vi "Telescope Move to RA and DEC.vi"(8 "error in (no error)":errorcluster, 10 "Object out":T1, 11 "Telescope in":refnum<class "Telescope.lvclass">) -> (0 "error out":errorcluster, 3 "Telescope out":refnum<class "Telescope.lvclass">)   [LabVIEW 2021, in "Telescope.lvclass"]
uses:
  Telescope.lvclass
  typedefs/CC cluster Object.ctl
  typedefs/CC cluster sidereal rate.ctl
  typedefs/CC cluster RA and DEC.ctl
  typedefs/cc cluster muRA muDEC.ctl
  CC cluster Telescope Offsets.ctl
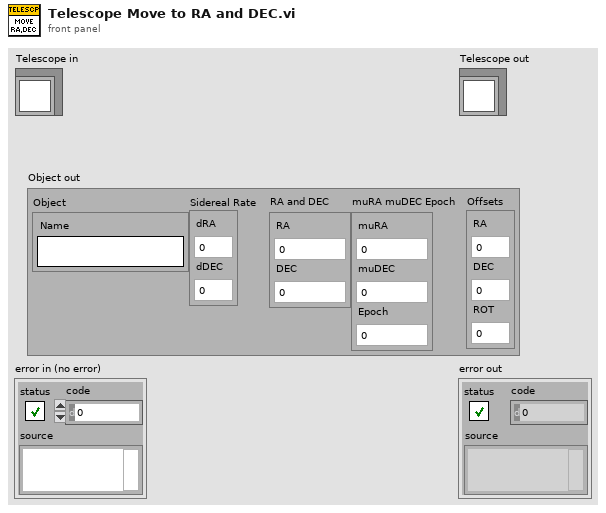
[diagram p1: front panel]
types:
  T1 = typedef "CC cluster Object.ctl" = cluster{"Object":cluster{"Name":string}, "Sidereal Rate":T2, "RA and DEC":T3, "muRA muDEC Epoch":T4, "Offsets":T5}
  T2 = typedef "CC cluster sidereal rate.ctl" = cluster{"dRA":dbl, "dDEC":dbl}
  T3 = typedef "CC cluster RA and DEC.ctl" = cluster{"RA":dbl, "DEC":dbl}
  T4 = typedef "cc cluster muRA muDEC.ctl" = cluster{"muRA":dbl, "muDEC":dbl, "Epoch":dbl}
  T5 = typedef "CC cluster Telescope Offsets.ctl" = cluster{"RA":dbl, "DEC":dbl, "ROT":dbl}
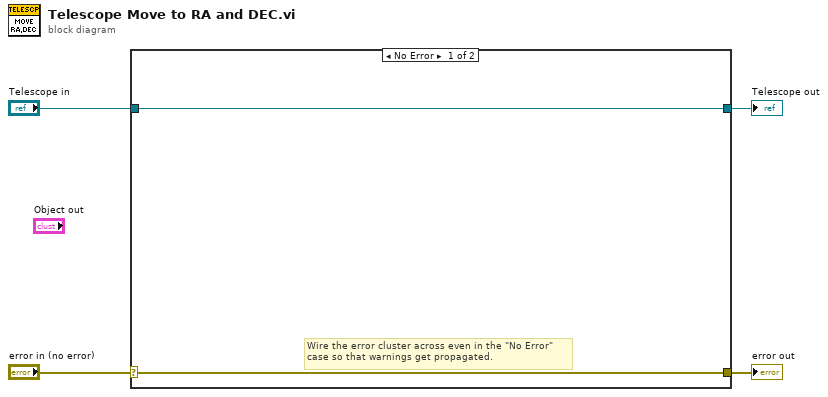
[diagram p0: block diagram]
diagram:
  n1 = case shown="No Error" "error in (no error)" {
    selector: "error in (no error)" -> [w5 w8]
    tunnel: [w5 w8] -> w3
    tunnel: [w6 w7] -> w1
    tunnel: "Telescope in" -> [w6 w7]
    frame No Error {
      # "Wire the error cluster across even in the \"No Error\"\ncase so that warnings get propagated."
    }
    frame Error {
    }
  }
  "error out" <- w3
  "Telescope out" <- w1
